vi "sbRIO.vi"() -> ()   [LabVIEW 2013]
uses:
  <vilib>/rvi/interface/nirviReadWriteControl/nirviReadWriteControl.xnode
  NiFpgaLv.dll
  <vilib>/Utility/error.llb/Error Cluster From Error Code.vi
  <vilib>/rvi/interface/Simulation/niFpgaSimulationCallBeginRW.vi
  <vilib>/rvi/errors/niLvFpgaAdjustHostInterfaceError.vi
  Helper Functions/ProcessorHelperFunctions.lvlib
  <vilib>/rvi/interface/nirviOpenFPGA/nirviOpenFPGA.xnode
  <vilib>/rvi/interface/nirviCloseFPGA/nirviCloseFPGA.xnode
  <vilib>/Platform/TimedLoop/XDataNode/wakeup.ctl
  <vilib>/Platform/TimedLoop/XDataNode/XDNodeRunTimeDep.lvlib
  <vilib>/Platform/TimedLoop/XDataNode/nitl_modes.ctl
  <vilib>/Platform/TimedLoop/XDataNode/timing_clust.ctl
  <vilib>/Platform/TimedLoop/XDataNode/XDataNode.xnode
  <vilib>/FPGAPlugInAG/Dynamic/niLvFpga_Close_Dynamic.vi
  FPGA Bitfiles/MidterminatorsSo_FPGATarget_FPGA_-ZxZV0zNGYo.lvbitx
  FPGA.vi
  <vilib>/FPGAPlugInAG/sbRIO-9642/niLvFpga_Open_sbRIO-9642.vi
  <vilib>/rvi/interface/common/dynamic/niFpgaDynamicAddResources.vi
panel:
  in  "Error Correction Speed":dbl=0.03
  out "Wheel Pos/Speed":picture
  out "Simulation Wheel Angles":dbl[](array[numeric])
  in  "Port":u16=2055 min=1025 step=1
  out "RX Data":T1
  in  "stop":bool
  in  "Manual Motor Control":bool=TRUE
  in  "Motor Number":u8
  out "Chassis Temp (C)":dbl
  out "E1":i64
  out "E3":i64
  out "E2":i64
  out "E4":i64
  out "A1":dbl
  out "A3":dbl
  out "A2":dbl
  out "A4":dbl
  out "T1":dbl
  out "T3":dbl
  out "T2":dbl
  out "T4":dbl
  in  "Calibration Mode":bool
  in  "Debug Mode":bool
  out "Wheel Target Angles":dbl[](array[numeric])
  out "Motor Output Values":u16[](array[slide]) scale=0.0..512.0
  in  "Offset1":i64
  in  "Offset3":i64
  in  "Offset2":i64
  in  "Offset4":i64
  # "Manual Motor Control"
  # "Encoder Count Pre Offset"
  # "Override All"
  # "Automatic\n  Control"
  # "Actual Wheel Angles"
  # "Target Wheel Angles"
  # "Wheel Calibration offsets"
  # "Debug"
  # "(ECS models physical \nparamaters of the robot)"
  # "Normal Operation"
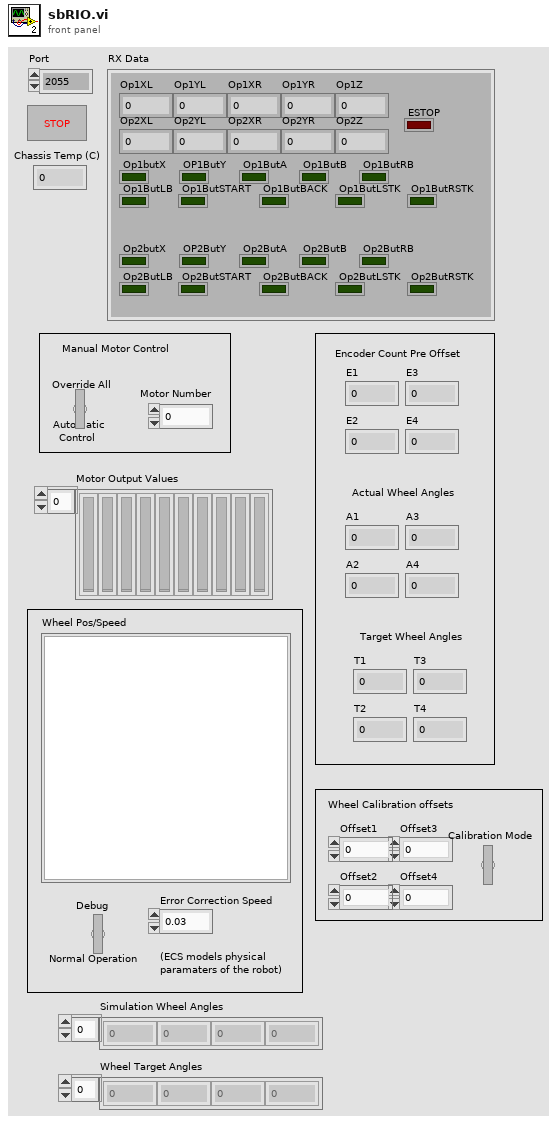
[diagram p1: front panel]
types:
  T1 = cluster{"Op2ButLSTK":bool, "Op2ButRSTK":bool, "Op1ButLSTK":bool, "Op1ButRSTK":bool, "Op1XL":i32, "Op1YL":i32, "Op1XR":i32, "Op1YR":i32, "Op1Z":i32, "Op2XL":i32, "Op2YL":i32, "Op2XR":i32, "Op2YR":i32, "Op2Z":i32, "ESTOP":bool, "Op1butX":bool, "OP1ButY":bool, "Op1ButA":bool, "Op1ButB":bool, "Op1ButRB":bool, "Op1ButLB":bool, "Op2butX":bool, "OP2ButY":bool, "Op2ButA":bool, "Op2ButB":bool, "Op2ButRB":bool, "Op2ButLB":bool, "Op2ButSTART":bool, "Op2ButBACK":bool, "Op1ButSTART":bool, "Op1ButBACK":bool}
  T2 = cluster{"Target Angles[0]":dbl, "Target Angles[1]":dbl, "Target Angles[2]":dbl, "Target Angles[3]":dbl}
  T3 = cluster{"MotorsOut[0]":u16, "MotorsOut[1]":u16, "MotorsOut[2]":u16, "MotorsOut[3]":u16, "MotorsOut[4]":u16, "MotorsOut[5]":u16, "MotorsOut[6]":u16, "MotorsOut[7]":u16, "MotorsOut[8]":u16, "MotorsOut[9]":u16, "MotorsOut[10]":u16, "MotorsOut[11]":u16}
  T4 = typedef "XDNodeRunTimeDep.lvlib/timing_clust.ctl" = cluster{"Expected End [f-1]":u64, "Actual End [f-1]":u64, "Finished Late? [f-1]":bool, "Expected End [i-1]":u64, "Actual End [i-1]":u64, "Finished Late? [i-1]":bool, "Expected Start [i]":u64, "Actual Start [i]":u64, "Expected Start [f]":u64, "Actual Start [f]":u64, "Source Name":string, "Structure Name":string, "Period":i64, "Deadline":i64, "Offset":i64, "Start":i64, "Priority":i32, "Timeout":i32, "Mode":T5, "Wakeup Reason":T6, "Error":errorcluster, "Source Type":string, "Secondary Source Type":string, "Global End Time":u64, "Global Start Time":u64, "Frame Duration":u64, "Iteration Duration":u64, "Assigned CPU":i32, "I/O Scan Engine Mode":u32}
  T5 = typedef "XDNodeRunTimeDep.lvlib/nitl_modes.ctl" = enum32{"No Change", "Process missed periods, maintain original phase", "Discard missed periods, maintain original phase", "Process missed periods, ignore original phase", "Discard missed periods, ignore original phase"}
  T6 = typedef "XDNodeRunTimeDep.lvlib/wakeup.ctl" = enum32{"Normal", "Aborted", "Asynchronous wakeup", "Timing source error", "Timed loop error", "Timeout"}
  T7 = cluster{"[0]":dbl, "[1]":dbl, "[2]":dbl, "[3]":dbl, "[4]":dbl, "[5]":dbl, "[6]":dbl, "[7]":dbl, "[8]":dbl}
  T8 = cluster{"[0]":u16, "[1]":u16, "[2]":u16, "[3]":u16}
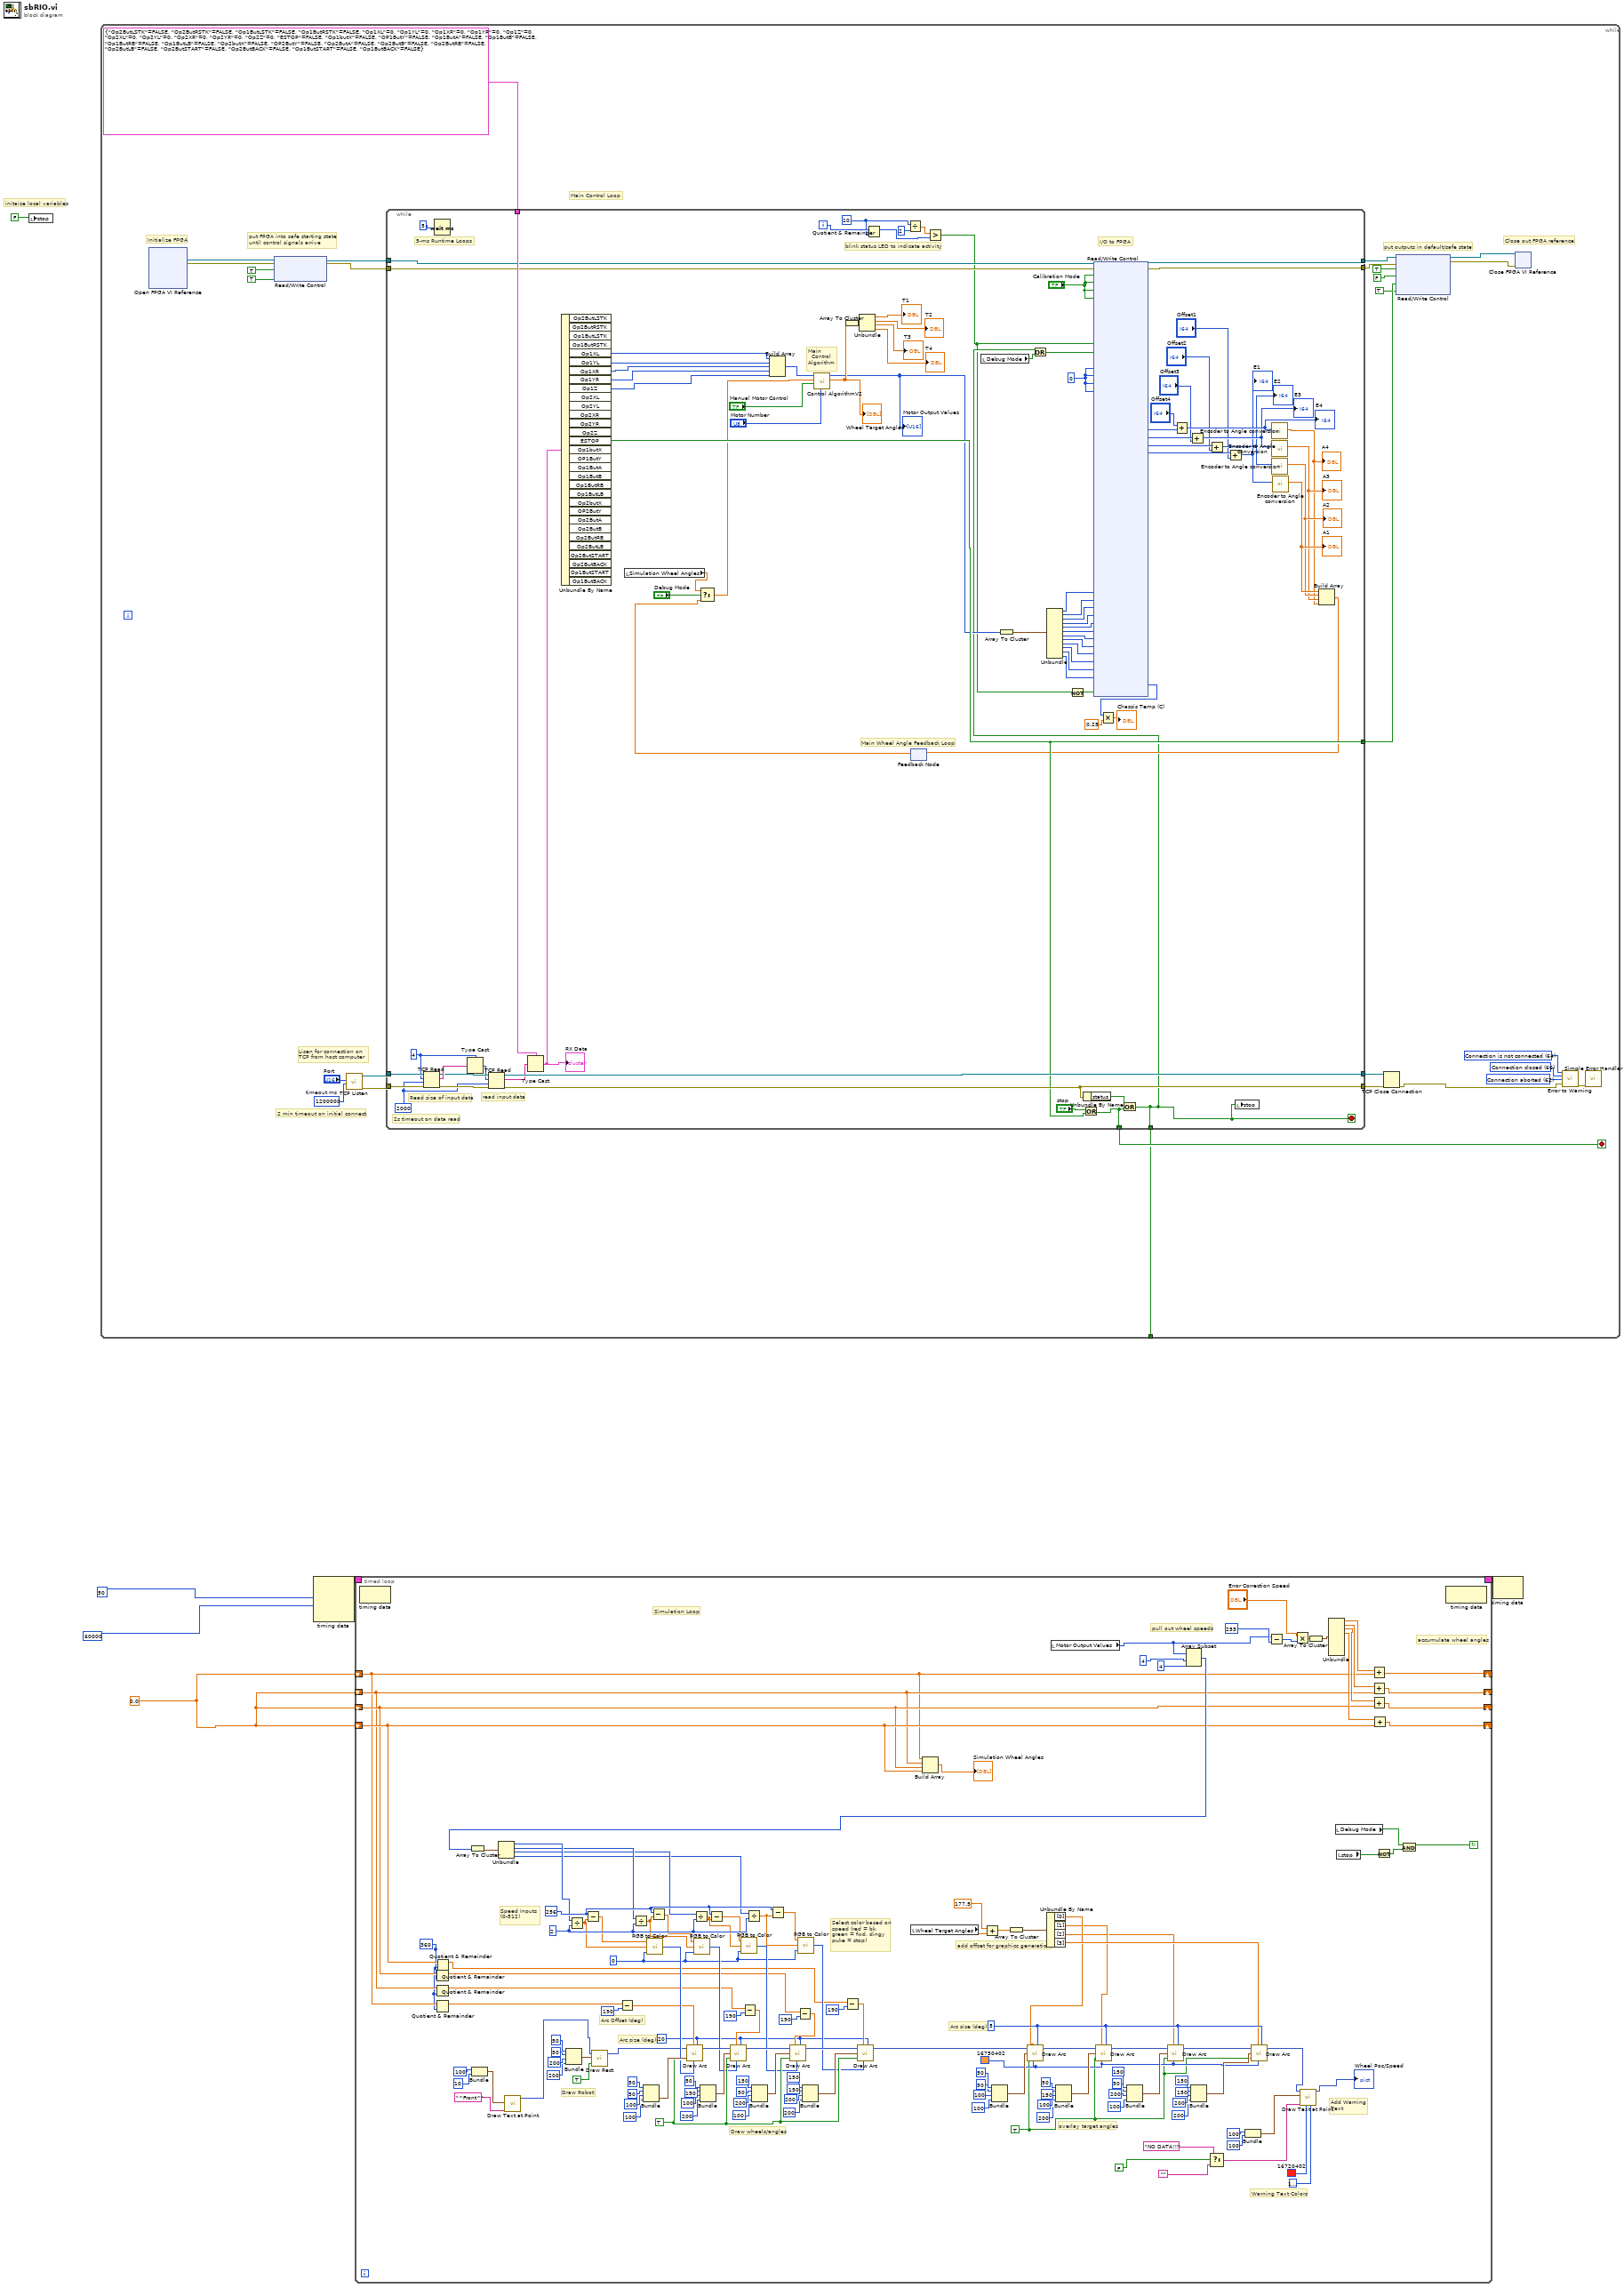
[diagram p0: block diagram]
diagram:
  w1 = 0.0
  # "initaize local variables"
  n1 = local write "stop"(FALSE) -> ()
  n2 = while {
    tunnel: [w7] -> _
    stop <- w8 stop-if-true
    w27 = 1200000  # timeout ms
    w31 = 62 items=["No Error", "Argument Error", "Memory Full", "Out of Zone", "End of File", "File Already Open", "Generic File IO Error", "File Not Found", "File Permission Error", "Disk Full", "Duplicate Path", "Too Many Files Open", "Not Enabled", "Resource File Not Found", "Cannot Add Resource", "Resource Not Found", "Image Not Found", "Image Memory Error", "Pen Does Not Exist", "Config Bad Type", "Config Token Not Found", "Config Parse Error", "Config Memory Error", "Bad External Code Format", "Bad External Code Offset", "External Code Not Present", "Null Window", "Destroy Window Mixup", "Null Menu", "Print Aborted", "Bad Print Record", "Print Driver Error", "Windows Error During Print", "Memory Error During Print", "Print Dialog Error", "Generic Print Error", "Invalid Device Refnum", "Device Not Found", "Device Parameter Error", "Device Unit Error", "Can't Open Device", "Device Call Aborted", "Generic Error", "Cancelled By User", "Object ID Too Low", "Object ID Too High", "Object Not In Heap", "Unknown Heap", "Bad DefProc ID", "DefProc Not In Table", "Message Out Of Range", "Null Method", "Unknown Message", "Manager Call Not Supported", "Bad address", "Connection In progress", "Connection timed out", "Connection is already in progress", "Network attribute not supported", "Network error", "Address in use", "System out of memory", "Connection aborted", "Connection refused", "Connection is not connected", "Connection is already connected", "Connection closed", "Initialize error (interapplication manager)", "Bad occurrence", "Wait on unbound occurrence handler", "Occurrence queue overflow", "Bad path", "Semaphore not signaled", "Unrecognized type (interapplication manager)"] ("1st Error to Convert")
    w32 = 66 items=["No Error", "Argument Error", "Memory Full", "Out of Zone", "End of File", "File Already Open", "Generic File IO Error", "File Not Found", "File Permission Error", "Disk Full", "Duplicate Path", "Too Many Files Open", "Not Enabled", "Resource File Not Found", "Cannot Add Resource", "Resource Not Found", "Image Not Found", "Image Memory Error", "Pen Does Not Exist", "Config Bad Type", "Config Token Not Found", "Config Parse Error", "Config Memory Error", "Bad External Code Format", "Bad External Code Offset", "External Code Not Present", "Null Window", "Destroy Window Mixup", "Null Menu", "Print Aborted", "Bad Print Record", "Print Driver Error", "Windows Error During Print", "Memory Error During Print", "Print Dialog Error", "Generic Print Error", "Invalid Device Refnum", "Device Not Found", "Device Parameter Error", "Device Unit Error", "Can't Open Device", "Device Call Aborted", "Generic Error", "Cancelled By User", "Object ID Too Low", "Object ID Too High", "Object Not In Heap", "Unknown Heap", "Bad DefProc ID", "DefProc Not In Table", "Message Out Of Range", "Null Method", "Unknown Message", "Manager Call Not Supported", "Bad address", "Connection In progress", "Connection timed out", "Connection is already in progress", "Network attribute not supported", "Network error", "Address in use", "System out of memory", "Connection aborted", "Connection refused", "Connection is not connected", "Connection is already connected", "Connection closed", "Initialize error (interapplication manager)", "Bad occurrence", "Wait on unbound occurrence handler", "Occurrence queue overflow", "Bad path", "Semaphore not signaled", "Unrecognized type (interapplication manager)"] ("1st Error to Convert")
    w33 = 64 items=["No Error", "Argument Error", "Memory Full", "Out of Zone", "End of File", "File Already Open", "Generic File IO Error", "File Not Found", "File Permission Error", "Disk Full", "Duplicate Path", "Too Many Files Open", "Not Enabled", "Resource File Not Found", "Cannot Add Resource", "Resource Not Found", "Image Not Found", "Image Memory Error", "Pen Does Not Exist", "Config Bad Type", "Config Token Not Found", "Config Parse Error", "Config Memory Error", "Bad External Code Format", "Bad External Code Offset", "External Code Not Present", "Null Window", "Destroy Window Mixup", "Null Menu", "Print Aborted", "Bad Print Record", "Print Driver Error", "Windows Error During Print", "Memory Error During Print", "Print Dialog Error", "Generic Print Error", "Invalid Device Refnum", "Device Not Found", "Device Parameter Error", "Device Unit Error", "Can't Open Device", "Device Call Aborted", "Generic Error", "Cancelled By User", "Object ID Too Low", "Object ID Too High", "Object Not In Heap", "Unknown Heap", "Bad DefProc ID", "DefProc Not In Table", "Message Out Of Range", "Null Method", "Unknown Message", "Manager Call Not Supported", "Bad address", "Connection In progress", "Connection timed out", "Connection is already in progress", "Network attribute not supported", "Network error", "Address in use", "System out of memory", "Connection aborted", "Connection refused", "Connection is not connected", "Connection is already connected", "Connection closed", "Initialize error (interapplication manager)", "Bad occurrence", "Wait on unbound occurrence handler", "Occurrence queue overflow", "Bad path", "Semaphore not signaled", "Unrecognized type (interapplication manager)"] ("1st Error to Convert")
    # "Main Control Loop"
    # "put FPGA into safe starting state\nuntil control signals arrive"
    # "put outputs in default/safe state"
    # "Close out FPGA reference"
    # "Initialize FPGA"
    # "2 min timeout on initial connect"
    # "Lisen for connection on \nTCP from host computer"
    n3 = xnode "Open FPGA VI Reference"() -> ("FPGA VI Reference Out"=w18:refnum<k20>, "error out"=w17:errorcluster)  [unwired: 2 in]
    n4 = xnode "Read/Write Control"("FPGA VI Reference In"=w18, "error in"=w17, "Stop All Motors"=TRUE, "Status LED"=TRUE) -> ("FPGA VI Reference Out"=w16:refnum<k20>, "error out"=w15:errorcluster)
    n5 = call <vilib>:"TCP Listen.vi"("timeout ms (wait forever: -1)"=w27, "port"="Port") -> ("error out"=w25:errorcluster, "connection ID"=w26:refnum<k5>)  [unwired: 5 in, 3 out]
    n6 = while {
      tunnel: w25 -> [w114]
      tunnel: w26 -> [w115]
      tunnel: [w116] -> w24
      tunnel: [w111] -> w23
      tunnel: T1 {"Op2ButLSTK"=FALSE, "Op2ButRSTK"=FALSE, "Op1ButLSTK"=FALSE, "Op1ButRSTK"=FALSE, "Op1XL"=0, "Op1YL"=0, "Op1XR"=0, "Op1YR"=0, "Op1Z"=0, "Op2XL"=0, "Op2YL"=0, "Op2XR"=0, "Op2YR"=0, "Op2Z"=0, "ESTOP"=FALSE, "Op1butX"=FALSE, "OP1ButY"=FALSE, "Op1ButA"=FALSE, "Op1ButB"=FALSE, "Op1ButRB"=FALSE, "Op1ButLB"=FALSE, "Op2butX"=FALSE, "OP2ButY"=FALSE, "Op2ButA"=FALSE, "Op2ButB"=FALSE, "Op2ButRB"=FALSE, "Op2ButLB"=FALSE, "Op2ButSTART"=FALSE, "Op2ButBACK"=FALSE, "Op1ButSTART"=FALSE, "Op1ButBACK"=FALSE} -> [w108]
      tunnel: w16 -> [w104]
      tunnel: w15 -> [w103]
      tunnel: [w102] -> w22
      tunnel: [w101] -> w21
      tunnel: [w95] -> w10
      tunnel: [w39] -> w7
      tunnel: [w46] -> w8
      i -> [w100]
      stop <- w39 stop-if-true
      w62 = 0
      w96 = 10
      w107 = 2000
      w112 = 4
      # "Main\n  Control\nAlgorithm"
      # "Main Wheel Angle Feedback Loop"
      # "blink status LED to indicate activity"
      # "I/O to FPGA"
      # "2s timeout on data read"
      # "read input data"
      # "Read size of input data"
      # "5-ms Runtime Loops"
      n7 = TCP Read(connection ID=w115, bytes to read=w112, error in (no error)=w114, 9:w107) -> (connection ID out=w119:refnum<k5>, data out=w120:string, error out=w118:errorcluster)  [unwired: 1 in]
      n8 = Wait (ms)(milliseconds to wait=u32 5) -> ()  [unwired: 1 out]
      n9 = Type Cast(type=w112, x=w120) -> (*(type *) &x=w117:i32)
      n10 = TCP Read(connection ID=w119, bytes to read=w117, error in (no error)=w118, 9:w107) -> (connection ID out=w116:refnum<k5>, data out=w113:string, error out=w111:errorcluster)  [unwired: 1 in]
      n11 = Type Cast(type=w108, x=w113) -> (*(type *) &x=w106:T1)
      "RX Data" <- w106
      n12 = Unbundle By Name(w106) -> ("Op1XL"=w44:i32, "Op1YL"=w43:i32, "Op1XR"=w42:i32, "Op1YR"=w41:i32, "Op1Z"=w40:i32, "ESTOP"=w95:bool)  [unwired: 25 out]
      n13 = local read "Simulation Wheel Angles"() -> (w59:dbl[])
      n14 = Build Array(w44, w43, w42, w41, w40) -> (w45:i32[])
      n15 = Quotient & Remainder(x=w100, y=w96) -> (x-y*floor(x/y)=w98:i32)  [unwired: 1 out]
      n16 = Divide(x=w96, y=2) -> (x/y=w97:dbl)
      n17 = feedback #1() -> (w60:dbl[])  [unwired: 1 in]
      n18 = Select(t=w59, s="Debug Mode", f=w60) -> (s? t:f=w57:dbl[])
      n19 = call "Control AlgorithmV2.vi"("Motor to Control"="Motor Number", "Manual Control"="Manual Motor Control", "Angles In"=w57, "JoystickIn"=w45) -> ("Target Angles"=w56:dbl[], "MotorsOut"=w55:u16[])  [unwired: 5 in]
      "Wheel Target Angles" <- w56
      "Motor Output Values" <- w55
      n20 = Array To Cluster(array=w56) -> (cluster=w77:T2)
      n21 = Unbundle(w77) -> ("Target Angles[0]"=→"T1":dbl, "Target Angles[1]"=→"T2":dbl, "Target Angles[2]"=→"T3":dbl, "Target Angles[3]"=→"T4":dbl)
      n22 = Greater?(x=w97, y=w98) -> (0:w35:bool)
      n23 = local read "Debug Mode"() -> (w37:bool)
      n24 = Array To Cluster(array=w55) -> (cluster=w83:T3)
      n25 = Unbundle(w83) -> ("MotorsOut[0]"=w93:u16, "MotorsOut[1]"=w92:u16, "MotorsOut[2]"=w91:u16, "MotorsOut[3]"=w90:u16, "MotorsOut[4]"=w89:u16, "MotorsOut[5]"=w88:u16, "MotorsOut[6]"=w87:u16, "MotorsOut[7]"=w86:u16, "MotorsOut[8]"=w85:u16, "MotorsOut[9]"=w84:u16, "MotorsOut[10]"=w82:u16, "MotorsOut[11]"=w81:u16)
      n26 = Not(x=w35) -> (.not. x?=w36:bool)
      n27 = Unbundle By Name(w111) -> ("status"=w110:bool)
      n28 = Or(x="stop", y=w95) -> (x .or. y?=w46:bool)
      n29 = Or(x=w110, y=w46) -> (x .or. y?=w39:bool)
      n30 = Or(x=w39, y=w37) -> (x .or. y?=w38:bool)
      n31 = xnode "Read/Write Control"("FPGA VI Reference In"=w104, "error in"=w103, "Cal. 4"="Calibration Mode", "Cal. 3"="Calibration Mode", "Cal.2"="Calibration Mode", "Cal.1"="Calibration Mode", "Status LED"=w35, "Stop All Motors"=w38, "Analog 3"=w62, "Analog 1"=w62, "Analog 4"=w62, "Analog 2"=w62, "Motor1"=w93, "Motor2"=w92, "Motor3"=w91, "Motor4"=w90, "Motor5"=w89, "Motor6"=w88, "Motor7"=w87, "Motor8"=w86, "Motor9"=w85, "Motor10"=w84, "Motor11"=w82, "Motor12"=w81, "FPGA LED"=w36) -> ("FPGA VI Reference Out"=w102:refnum<k20>, "error out"=w101:errorcluster, "Encoder4"=w72:i64, "Encoder3"=w71:i64, "Encoder2"=w70:i64, "Encoder1"=w69:i64, "Chasis Temp"=w78:i16)  [unwired: 14 in, 13 out]
      n32 = Multiply(x=w78, y=0.25) -> (x*y=→"Chassis Temp (C)":dbl)
      n33 = Add(x="Offset4", y=w72) -> (x+y=w54:i64)
      "E4" <- w54
      n34 = Add(x=w71, y="Offset3") -> (x+y=w52:i64)
      "E3" <- w52
      n35 = Add(x=w70, y="Offset2") -> (x+y=w51:i64)
      "E2" <- w51
      n36 = Add(x=w69, y="Offset1") -> (x+y=w50:i64)
      "E1" <- w50
      n37 = local write "stop"(w39) -> ()
      n38 = call "Encoder to Angle conversion.vi"("Input"=w54) -> ("Output"=w65:dbl)  [unwired: 10 in]
      "A4" <- w65
      n39 = call "Encoder to Angle conversion.vi"("Input"=w52) -> ("Output"=w66:dbl)  [unwired: 10 in]
      "A3" <- w66
      n40 = call "Encoder to Angle conversion.vi"("Input"=w51) -> ("Output"=w67:dbl)  [unwired: 10 in]
      "A2" <- w67
      n41 = call "Encoder to Angle conversion.vi"("Input"=w50) -> ("Output"=w68:dbl)  [unwired: 10 in]
      "A1" <- w68
      n42 = Build Array(w68, w67, w66, w65) -> (w64:dbl[])
      n43 = feedback-in #1(w64) -> ()
    }
    n44 = TCP Close Connection(connection ID=w24, error in (no error)=w23) -> (error out=w29:errorcluster)  [unwired: 1 in, 1 out]
    n45 = xnode "Read/Write Control"("FPGA VI Reference In"=w22, "error in"=w21, "Stop All Motors"=TRUE, "Status LED"=FALSE, "Emergency Stop"=w10, "Halt Execution"=TRUE) -> ("FPGA VI Reference Out"=w20:refnum<k20>, "error out"=w13:errorcluster)
    n46 = xnode "Close FPGA VI Reference"("FPGA VI Reference In"=w20, "error in"=w13) -> ()  [unwired: 1 out]
    n47 = call <vilib>:"Error to Warning.vi"("1st Error to Convert"=w33, "2nd Error to Convert"=w32, "3rd Error to Convert"=w31, "error in"=w29) -> ("warning out"=w34:errorcluster)  [unwired: 11 in]
    n48 = call <vilib>:"Simple Error Handler.vi"("error in (no error)"=w34) -> ()  [unwired: 4 in, 5 out]
  }
  n49 = node-c288(50, 60000) -> (w5:T4)  [unwired: 2 in]
  n50 = timed-loop {
    timing: w5 -> [_]
    timing-out: [_] -> w4
    shift-right: [w257] -> _
    shift-left: w1 -> [w129]
    shift-right: [w256] -> _
    shift-left: w1 -> [w131]
    shift-right: [w258] -> _
    shift-left: w1 -> [w127]
    shift-right: [w259] -> _
    shift-left: w1 -> [w125]
    stop <- w123 continue-if-true
    w124 = 360
    w151 = TRUE
    w154 = 5
    w155 = u32 16750402
    w195 = 20
    w197 = 0
    w213 = 2
    w214 = 256
    w226 = TRUE
    # "Simulation Loop"
    # "add offset for graphics generation"
    # "pull out wheel speeds"
    # "Arc size (deg)"
    # "overlay target angles"
    # "Add Warning\nText"
    # "Warning Text Colors"
    # "Arc Offset (deg)"
    # "Arc size (deg)"
    # "Speed Inputs (0-512)"
    # "Draw wheels/angles"
    # "Select color based on speed (red = bk, green = fwd, dingy puke = stop)"
    # "Draw Robot"
    # "accumulate wheel angles"
    n51 = node-c288() -> ()  [unwired: 1 in, 1 out]
    n52 = Quotient & Remainder(x=w129, y=w124) -> (x-y*floor(x/y)=w130:dbl)  [unwired: 1 out]
    n53 = Quotient & Remainder(x=w127, y=w124) -> (x-y*floor(x/y)=w128:dbl)  [unwired: 1 out]
    n54 = Quotient & Remainder(x=w125, y=w124) -> (x-y*floor(x/y)=w126:dbl)  [unwired: 1 out]
    n55 = Quotient & Remainder(x=w131, y=w124) -> (x-y*floor(x/y)=w132:dbl)  [unwired: 1 out]
    n56 = Bundle(100, 10) -> (w190:cluster{i32, i32})  [unwired: 1 in]
    n57 = call <vilib>:"Draw Text at Point.vi"("text"="^Front^", "origin"=w190) -> ("new picture"=w194:picture)  [unwired: 8 in, 1 out]
    n58 = Bundle(50, 50, 200, 200) -> (w217:cluster{i32, i32, i32, i32})  [unwired: 1 in]
    n59 = call <vilib>:"Draw Rect.vi"("picture"=w194, "rect"=w217, "fill?(F)"=TRUE) -> ("new picture"=w215:picture)  [unwired: 6 in]
    n60 = Subtract(x=w126, y=190) -> (x-y=w203:dbl)
    n61 = Bundle(50, 50, 100, 100) -> (w243:cluster{i32, i32, i32, i32})  [unwired: 1 in]
    n62 = Bundle(50, 150, 100, 200) -> (w229:cluster{i32, i32, i32, i32})  [unwired: 1 in]
    n63 = Subtract(x=w128, y=190) -> (x-y=w199:dbl)
    n64 = Bundle(150, 50, 200, 100) -> (w228:cluster{i32, i32, i32, i32})  [unwired: 1 in]
    n65 = Subtract(x=w130, y=190) -> (x-y=w198:dbl)
    n66 = Bundle(150, 150, 200, 200) -> (w227:cluster{i32, i32, i32, i32})  [unwired: 1 in]
    n67 = Subtract(x=w132, y=190) -> (x-y=w196:dbl)
    n68 = local read "Wheel Target Angles"() -> (w140:dbl[])
    n69 = Build Array(w125, w127, w129, w131) -> (→"Simulation Wheel Angles":dbl[])
    n70 = Add(x=177.5, y=w140) -> (x+y=w137:dbl[])
    n71 = Bundle(50, 50, 100, 100) -> (w173:cluster{i32, i32, i32, i32})  [unwired: 1 in]
    n72 = Array To Cluster(array=w137) -> (cluster=w153:T7)
    n73 = Unbundle By Name(w153) -> ("[0]"=w135:dbl, "[1]"=w134:dbl, "[2]"=w133:dbl, "[3]"=w152:dbl)
    n74 = local read "Motor Output Values"() -> (w141:u16[])
    n75 = Bundle(50, 150, 100, 200) -> (w167:cluster{i32, i32, i32, i32})  [unwired: 1 in]
    n76 = Bundle(150, 50, 200, 100) -> (w162:cluster{i32, i32, i32, i32})  [unwired: 1 in]
    n77 = Array Subset(array=w141, index=4, length=4) -> (w146:u16[])
    n78 = Array To Cluster(array=w146) -> (cluster=w147:T8)
    n79 = Unbundle(w147) -> ("[0]"=w145:u16, "[1]"=w144:u16, "[2]"=w143:u16, "[3]"=w142:u16)
    n80 = Divide(x=w145, y=w213) -> (x/y=w212:dbl)
    n81 = Subtract(x=w214, y=w212) -> (x-y=w209:dbl)
    n82 = Divide(x=w144, y=w213) -> (x/y=w211:dbl)
    n83 = call <vilib>:"RGB to Color.vi"("B"=w197, "G"=w212, "R"=w209) -> ("Color"=w225:u32)
    n84 = Subtract(x=w214, y=w211) -> (x-y=w208:dbl)
    n85 = call <vilib>:"Draw Arc.vi"("picture"=w215, "start angle[degrees]"=w203, "rect"=w243, "fill?(F)"=w226, "color(black)"=w225, "arc size[degrees]"=w195) -> ("new picture"=w249:picture)  [unwired: 3 in]
    n86 = Divide(x=w143, y=w213) -> (x/y=w207:dbl)
    n87 = call <vilib>:"RGB to Color.vi"("B"=w197, "G"=w211, "R"=w208) -> ("Color"=w224:u32)
    n88 = Subtract(x=w214, y=w207) -> (x-y=w206:dbl)
    n89 = call <vilib>:"Draw Arc.vi"("picture"=w249, "start angle[degrees]"=w199, "rect"=w229, "fill?(F)"=w226, "color(black)"=w224, "arc size[degrees]"=w195) -> ("new picture"=w248:picture)  [unwired: 3 in]
    n90 = call <vilib>:"RGB to Color.vi"("B"=w197, "G"=w207, "R"=w206) -> ("Color"=w223:u32)
    n91 = Divide(x=w142, y=w213) -> (x/y=w210:dbl)
    n92 = Subtract(x=w214, y=w210) -> (x-y=w205:dbl)
    n93 = call <vilib>:"Draw Arc.vi"("picture"=w248, "start angle[degrees]"=w198, "rect"=w228, "fill?(F)"=w226, "color(black)"=w223, "arc size[degrees]"=w195) -> ("new picture"=w247:picture)  [unwired: 3 in]
    n94 = call <vilib>:"RGB to Color.vi"("B"=w197, "G"=w210, "R"=w205) -> ("Color"=w222:u32)
    n95 = call <vilib>:"Draw Arc.vi"("picture"=w247, "start angle[degrees]"=w196, "rect"=w227, "fill?(F)"=w226, "color(black)"=w222, "arc size[degrees]"=w195) -> ("new picture"=w179:picture)  [unwired: 3 in]
    n96 = call <vilib>:"Draw Arc.vi"("picture"=w179, "start angle[degrees]"=w135, "rect"=w173, "fill?(F)"=w151, "color(black)"=w155, "arc size[degrees]"=w154) -> ("new picture"=w178:picture)  [unwired: 3 in]
    n97 = call <vilib>:"Draw Arc.vi"("picture"=w178, "start angle[degrees]"=w134, "rect"=w167, "fill?(F)"=w151, "color(black)"=w155, "arc size[degrees]"=w154) -> ("new picture"=w161:picture)  [unwired: 3 in]
    n98 = call <vilib>:"Draw Arc.vi"("picture"=w161, "start angle[degrees]"=w133, "rect"=w162, "fill?(F)"=w151, "color(black)"=w155, "arc size[degrees]"=w154) -> ("new picture"=w177:picture)  [unwired: 3 in]
    n99 = Bundle(150, 150, 200, 200) -> (w156:cluster{i32, i32, i32, i32})  [unwired: 1 in]
    n100 = Select(t="NO DATA!!!", s=FALSE, f="") -> (s? t:f=w183:string)
    n101 = Bundle(100, 100) -> (w186:cluster{i32, i32})  [unwired: 1 in]
    n102 = call <vilib>:"Draw Arc.vi"("picture"=w177, "start angle[degrees]"=w152, "rect"=w156, "fill?(F)"=w151, "color(black)"=w155, "arc size[degrees]"=w154) -> ("new picture"=w180:picture)  [unwired: 3 in]
    n103 = Subtract(x=w141, y=255) -> (x-y=w261:i32[])
    n104 = Multiply(x="Error Correction Speed", y=w261) -> (x*y=w255:dbl[])
    n105 = call <vilib>:"Draw Text at Point.vi"("BG color(transparent)"=u32 16777216, "text color(black)"=u32 16720402, "text"=w183, "origin"=w186, "picture"=w180) -> ("new picture"=→"Wheel Pos/Speed":picture)  [unwired: 5 in, 1 out]
    n106 = Array To Cluster(array=w255) -> (cluster=w260:T7)
    n107 = Unbundle(w260) -> ("[0]"=w253:dbl, "[1]"=w252:dbl, "[2]"=w251:dbl, "[3]"=w250:dbl)  [unwired: 5 out]
    n108 = local read "Debug Mode"() -> (w138:bool)
    n109 = local read "stop"() -> (w121:bool)
    n110 = Add(x=w253, y=w125) -> (x+y=w259:dbl)
    n111 = Add(x=w252, y=w127) -> (x+y=w258:dbl)
    n112 = Add(x=w251, y=w129) -> (x+y=w257:dbl)
    n113 = Add(x=w250, y=w131) -> (x+y=w256:dbl)
    n114 = Not(x=w121) -> (.not. x?=w122:bool)
    n115 = And(x=w138, y=w122) -> (x .and. y?=w123:bool)
    n116 = node-c288() -> ()  [unwired: 1 in, 1 out]
  }
  n117 = node-c288(w4) -> ()  [unwired: 1 out]
